vi "Read Velocity.vi"(8 "error in":errorcluster, 11 "Mover in":refnum<class "Mover.lvclass">) -> (0 "error out":errorcluster, 2 "Velocity PVector":refnum<class "PVector.lvclass">, 3 "Mover out":refnum<class "Mover.lvclass">)   [LabVIEW 2016, in "Mover.lvclass"]
uses:
  Mover.lvclass
  PVector/PVector.lvclass
  Mover.lvclass/Mover.ctl
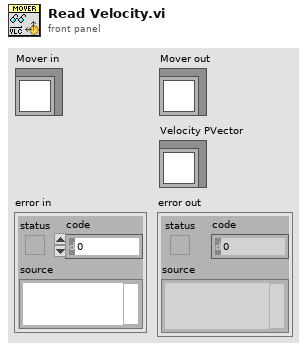
[diagram p1: front panel]
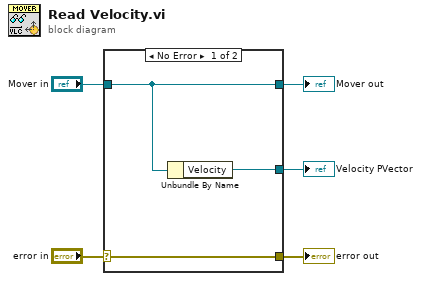
[diagram p0: block diagram]
diagram:
  n1 = case shown="No Error" "error in" {
    selector: "error in" -> [w8 w9]
    tunnel: [w8 w9] -> w4
    tunnel: [w7 w10] -> w2
    tunnel: "Mover in" -> [w7 w10]
    tunnel: [w6 _] -> w1
    frame No Error {
      n2 = Unbundle By Name(w7) -> ("Velocity"=w6:refnum<class "PVector.lvclass">)
    }
    frame Error {
    }
  }
  "error out" <- w4
  "Mover out" <- w2
  "Velocity PVector" <- w1
